vi "Make Path Rear First.vi"(0 "Segments in":T1[](array[typedef]), 11 "error in (no error)":errorcluster) -> (4 "Segments out":T1[](array[typedef]), 15 "error out":errorcluster)   [LabVIEW 2017]
uses:
  VIs/Segment.ctl
  Pathfinder.lvlib
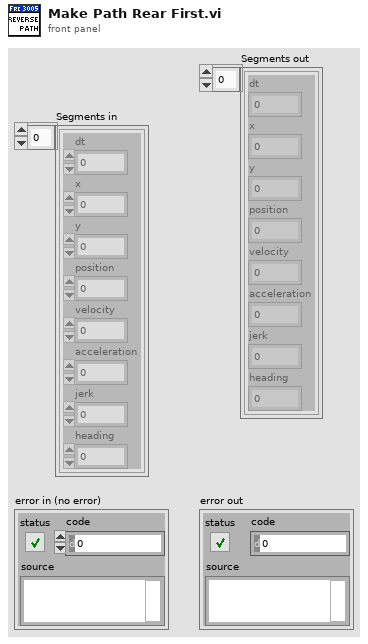
[diagram p1: front panel]
types:
  T1 = typedef "Pathfinder.lvlib/Segment.ctl" = cluster{"dt":dbl, "x":dbl, "y":dbl, "position":dbl, "velocity":dbl, "acceleration":dbl, "jerk":dbl, "heading":dbl}
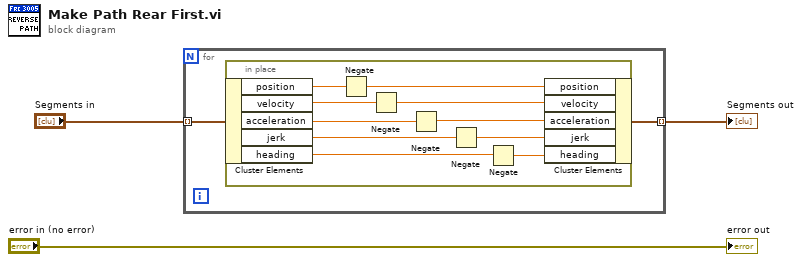
[diagram p0: block diagram]
diagram:
  n1 = for {
    tunnel: "Segments in" -> [w5] mode=indexing
    tunnel: [w4] -> w2 mode=indexing
    n2 = in-place {
      n3 = in-place-cluster #1(w5) -> ("position"=w15:dbl, "velocity"=w13:dbl, "acceleration"=w11:dbl, "jerk"=w9:dbl, "heading"=w7:dbl)
      n4 = Negate(x=w15) -> (-x=w14:dbl)
      n5 = Negate(x=w13) -> (-x=w12:dbl)
      n6 = Negate(x=w11) -> (-x=w10:dbl)
      n7 = Negate(x=w9) -> (-x=w6:dbl)
      n8 = Negate(x=w7) -> (-x=w8:dbl)
      n9 = in-place-cluster #1("position"=w14, "velocity"=w12, "acceleration"=w10, "jerk"=w6, "heading"=w8) -> (w4:T1)
    }
  }
  "Segments out" <- w2
  "error out" <- "error in (no error)"
